vi "largeP_READ.vi"() -> ()   [LabVIEW 2009]
panel:
  out "value":dbl[](graph)
  out "size(s)":i32
  out "error out":errorcluster
  out "data out":string
  out "DATA Connection listener ID":refnum<k5>
  out "*(type *) &x":i32
  out "data out 3":string
  in  "STOP":refnum<vi>
  # "800004"
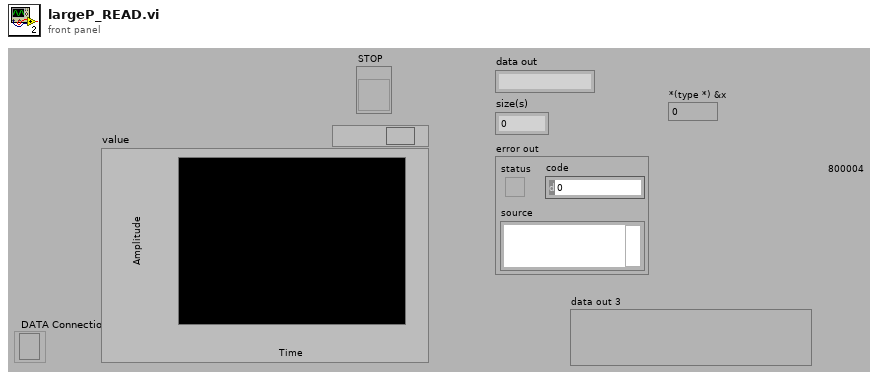
[diagram p1: front panel]
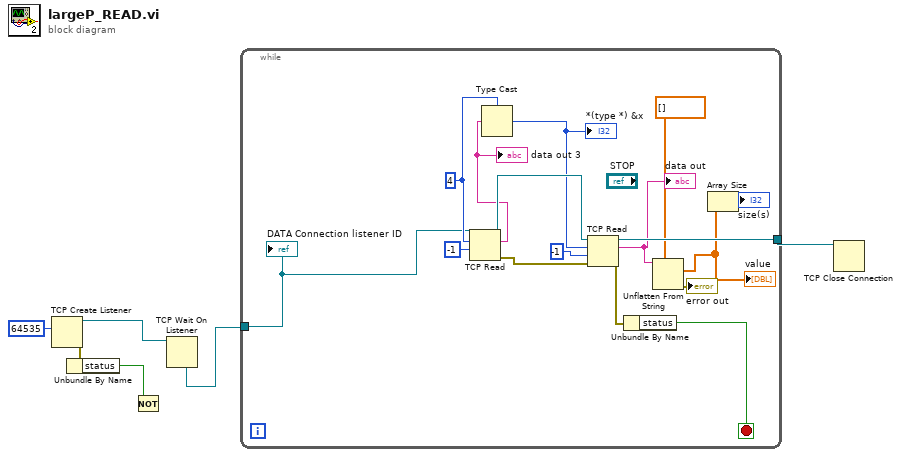
[diagram p0: block diagram]
diagram:
  n1 = TCP Create Listener(10:u16 64535 ("DATA port")) -> (0:w4:errorcluster, 3:w2:refnum<k5>)  [unwired: 3 in, 2 out]
  n2 = Unbundle By Name(w4) -> ("status"=w3:bool)
  n3 = Not(x=w3) -> ()  [unwired: 1 out]
  n4 = TCP Wait On Listener(11:w2) -> (4:w1:refnum<k5>)  [unwired: 1 in, 6 out]
  n5 = while {
    tunnel: w1 -> [w14]
    tunnel: [w13] -> w6
    stop <- w15 stop-if-true
    w18 = 4
    n6 = TCP Read(connection ID=w14, bytes to read=w18, 9:-1 ("timeout ms (25000)")) -> (connection ID out=w21:refnum<k5>, data out=w19:string, error out=w22:errorcluster)  [unwired: 2 in]
    "data out 3" <- w19
    n7 = Type Cast(type=w18, x=w19) -> (*(type *) &x=w12:i32)
    "*(type *) &x" <- w12
    n8 = TCP Read(connection ID=w21, bytes to read=w12, error in (no error)=w22, 9:-1) -> (connection ID out=w13:refnum<k5>, data out=w11:string, error out=w16:errorcluster)  [unwired: 1 out]
    "data out" <- w11
    n9 = Unbundle By Name(w16) -> ("status"=w15:bool)
    n10 = Unflatten From String(type=dbl[] [], binary string=w11) -> (value=w8:dbl[], error out=→"error out":errorcluster)  [unwired: 3 in, 1 out]
    "value" <- w8
    n11 = Array Size(array=w8) -> (size(s)=→"size(s)":i32)
    "DATA Connection listener ID" <- w14
  }
  n12 = TCP Close Connection(connection ID=w6) -> ()  [unwired: 2 in, 2 out]
